vi "Elapsed Time.vi"() -> (0 "Elapsed Time (sec)":dbl format="%.2f")   [LabVIEW 2012]
doc: "NOTE: This VI was built to be used in conjunction with either Automatic VI Server Connection Polling.vi or Manual VI Server Connection Polling.vi. For instructions, see either of these VI Server Connection Polling VIs. When run, this VI will keep track of its elapsed time."
uses:
  Instance           2 43Saved   VI Server Connection Polling Target .vi
  Instance           1 43Saved   VI Server Connection Polling Target .vi
panel:
  out "Elapsed Time (sec) 2":dbl format="%.2f"
  in  "RESET":bool
  in  "Numeric":dbl
  out "Date & Time":string
  out "Boolean":bool
  out "Start Time":string
  out "Elapsed Time (d hh:mm:ss)":string
  in  "stop":bool
  # "NOTE: This VI was built to be used in conjunction with either Automatic VI Server Connection Polling.vi or Manual VI Server Connection Polling.vi.  For instructions, see either of these examples.  When run, this VI will keep track of its elapsed time."
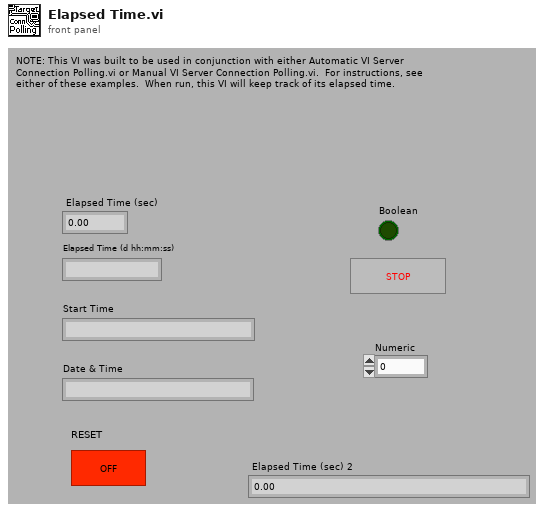
[diagram p1: front panel]
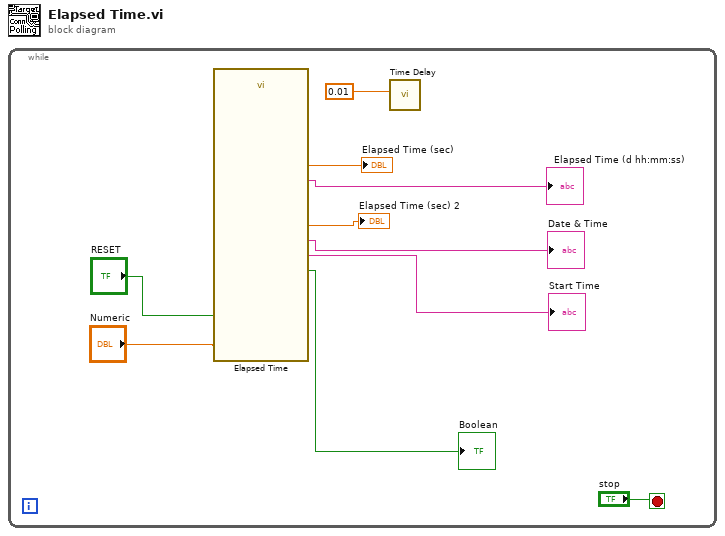
[diagram p0: block diagram]
diagram:
  n1 = while {
    stop <- "stop" stop-if-true
    n2 = call "Elapsed Time"("Time Target (s)"="Numeric", "Reset"="RESET") -> ("Start Time Text"=→"Start Time":string, "Present (s)"=→"Elapsed Time (sec) 2":dbl, "Present Text"=→"Date & Time":string, "Elapsed Time (s)"=→"Elapsed Time (sec)":dbl, "Time has Elapsed"=→"Boolean":bool, "Elapsed Time Text"=→"Elapsed Time (d hh:mm:ss)":string)  [unwired: 10 in, 2 out]
    n3 = call "Time Delay"("Delay Time (s)"=0.01) -> ()  [unwired: 10 in, 1 out]
  }
